vi "Write Keys.vi"(8 "error in":errorcluster, 10 "Keys":string[](array[string]), 11 "Object Entry in":refnum<class "Object Entry.lvclass">) -> (0 "error out":errorcluster, 3 "Object Entry out":refnum<class "Object Entry.lvclass">)   [LabVIEW 2024, in "EDS.lvlib" / "Object Entry.lvclass"]
uses:
  Object Entry.lvclass
  Object Entry.lvclass/Object Entry.ctl
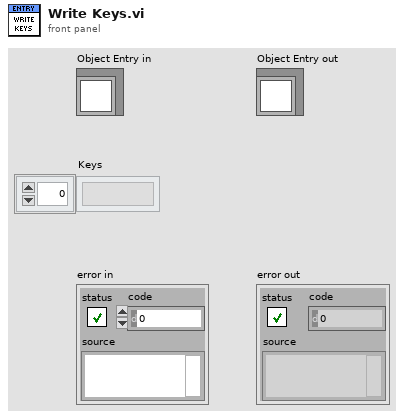
[diagram p1: front panel]
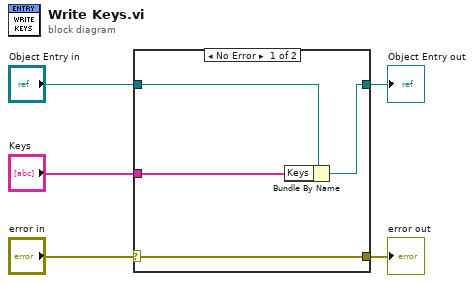
[diagram p0: block diagram]
diagram:
  n1 = case shown="No Error" "error in" {
    selector: "error in" -> [w9 w10]
    tunnel: [w9 w10] -> w4
    tunnel: [w7 w11] -> w2
    tunnel: "Object Entry in" -> [w8 w11]
    tunnel: "Keys" -> [w6 _]
    frame No Error {
      n2 = Bundle By Name(cluster=w8, "Keys"=w6) -> (w7:refnum<class "Object Entry.lvclass">)
    }
    frame Error {
    }
  }
  "error out" <- w4
  "Object Entry out" <- w2
